vi "Swap Controllers.vi"(8 "error in (no error)":errorcluster, 10 "Cooler Controller":refnum<class "Cooler Controller.lvclass">, 11 "Air Cooler Application in":refnum<class "Air Cooler Application.lvclass">) -> (0 "error out":errorcluster, 3 "Air Cooler Application out":refnum<class "Air Cooler Application.lvclass">)   [LabVIEW 2018, in "Air Cooler Application.lvlib" / "Air Cooler Application.lvclass"]
doc: "This VI changes which controller actor is currently running. The input controller will be launched and the existing controller will be stopped. The cooler continues running uninterrupted during this transition."
uses:
  Air Cooler Application.lvclass
  C:/Program Files (x86)/National Instruments/LabVIEW 2018/vi.lib/ActorFramework/Actor/Actor.lvclass
  Cooler Controller/Cooler Controller/Cooler Controller.lvclass
  <vilib>/ActorFramework/Message Enqueuer/Message Enqueuer.lvclass
  <vilib>/ActorFramework/Message Enqueuer/Message Priority.ctl
  Air Cooler Application.lvclass/Air Cooler Application.ctl
  Cooler Controller/Write Cooler Enqueuer Msg/Write Cooler Enqueuer Msg.lvclass/Write Cooler Enqueuer Msg.ctl
  <vilib>/ActorFramework/Message Enqueuer/Message Enqueuer.lvclass/Message Enqueuer.ctl
  Cooler/Write Controller Enqueuer Msg/Write Controller Enqueuer Msg.lvclass/Write Controller Enqueuer Msg.ctl
  <vilib>/ActorFramework/Message Enqueuer/Enqueue.vi
  Cooler Controller/Write Cooler Enqueuer Msg/Write Cooler Enqueuer Msg.lvclass
  C:/Program Files (x86)/National Instruments/LabVIEW 2018/vi.lib/ActorFramework/Message/Message.lvclass
  Cooler/Write Controller Enqueuer Msg/Write Controller Enqueuer Msg.lvclass
  <vilib>/ActorFramework/Stop Msg/Stop Msg.lvclass
  <vilib>/ActorFramework/Message Priority Queue/Priority Enqueue.vi
  <vilib>/ActorFramework/Actor/Actor.lvclass
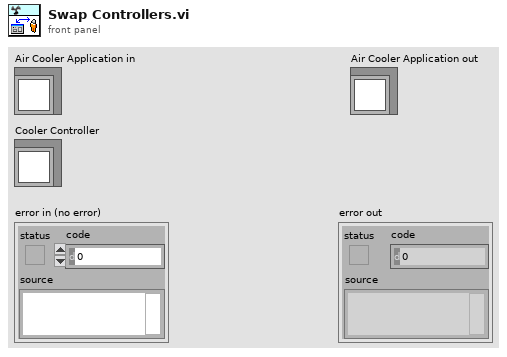
[diagram p1: front panel]
types:
  T1 = typedef "Actor Framework.lvlib/Message Enqueuer.lvclass/Message Priority.ctl" = enum16{"Low", "Normal", "High"}
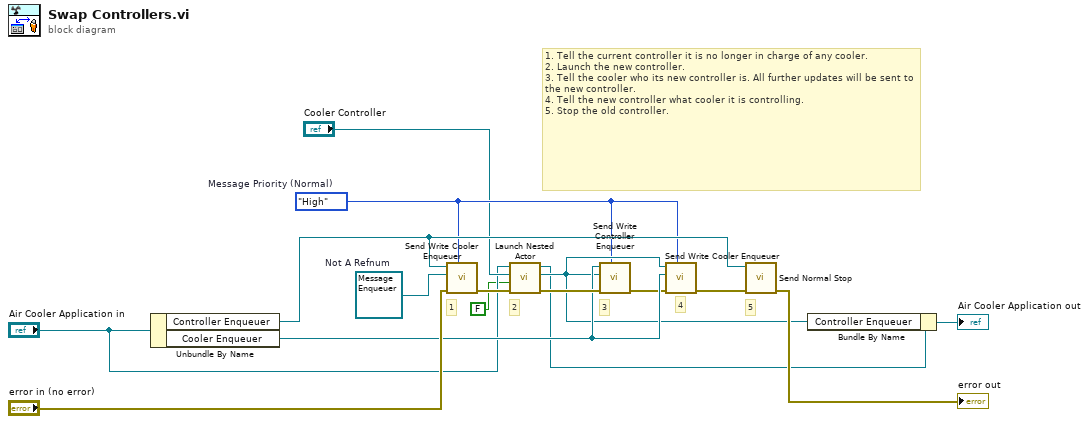
[diagram p0: block diagram]
diagram:
  w5 = Message_Priority."High"  # Message Priority (Normal)
  w12 = refnum<class "Message Enqueuer.lvclass"> refnum  # Not A Refnum
  # "4"
  # "1. Tell the current controller it is no longer in charge of any cooler.\n2. Launch the new controller. \n3. Tell the cooler who its new controller is. All further updates will be sent to the new controller.\n4. Tell the new controller what cooler it is controlling.\n5. Stop the old controller."
  # "5"
  # "3"
  # "2"
  # "1"
  n1 = Unbundle By Name("Air Cooler Application in") -> ("Controller Enqueuer"=w10:refnum<class "Message Enqueuer.lvclass">, "Cooler Enqueuer"=w9:refnum<class "Message Enqueuer.lvclass">)
  n2 = call "Send Write Cooler Enqueuer.vi"("Message Priority (Normal)"=w5, "error in (no error)"="error in (no error)", "Cooler Enqueuer"=w12, "Message Enqueuer"=w10) -> ("error out"=w13:errorcluster)  [unwired: 7 in]
  n3 = call <vilib>:"Launch Nested Actor.vi"("error in (no error)"=w13, "Auto-stop? (T)"=FALSE, "Nested Actor"="Cooler Controller", "Caller Actor in"="Air Cooler Application in") -> ("error out"=w11:errorcluster, "Nested Actor's Enqueuer"=w8:refnum<class "Message Enqueuer.lvclass">, "Caller Actor out"=w2:refnum<class "Air Cooler Application.lvclass">)  [unwired: 5 in]
  n4 = call "Send Write Controller Enqueuer.vi"("Message Priority (Normal)"=w5, "error in (no error)"=w11, "Controller Enqueuer"=w8, "Message Enqueuer"=w9) -> ("error out"=w7:errorcluster)  [unwired: 7 in]
  n5 = call "Send Write Cooler Enqueuer.vi"("Message Priority (Normal)"=w5, "error in (no error)"=w7, "Cooler Enqueuer"=w9, "Message Enqueuer"=w8) -> ("error out"=w6:errorcluster)  [unwired: 7 in]
  n6 = call <vilib>:"Send Normal Stop.vi"("error in (no error)"=w6, "Message Enqueuer"=w10) -> ("error out"=→"error out":errorcluster)  [unwired: 9 in]
  n7 = Bundle By Name(cluster=w2, "Controller Enqueuer"=w8) -> (→"Air Cooler Application out":refnum<class "Air Cooler Application.lvclass">)
